vi "Get DAQ Time Array from Waveform.vi"(8 "error in (no error)":errorcluster, 9 "DAQ dt":dbl format="%#_13g", 10 "DAQ Average Number of Points":dbl format="%#_13g", 11 "DAQ Number of Samples":dbl) -> (0 "error out":errorcluster, 3 "Time Axis":dbl[](array[numeric]))   [LabVIEW 2017, in "File IO.lvlib"]
uses:
  File IO.lvlib
  <vilib>/Analysis/2dsp.llb/Decimate (single shot, DBL).vi
  <vilib>/Analysis/NI_AALPro.lvlib
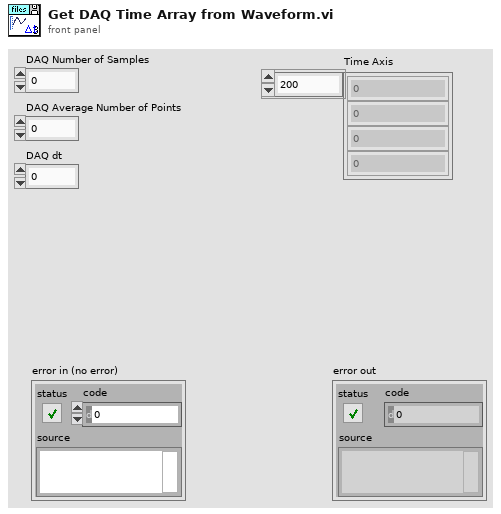
[diagram p1: front panel]
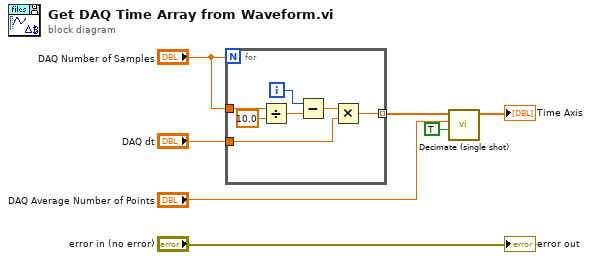
[diagram p0: block diagram]
diagram:
  n1 = for {
    N: "DAQ Number of Samples" -> [_]
    tunnel: "DAQ Number of Samples" -> [w14]
    tunnel: [w9] -> w7 mode=indexing
    tunnel: "DAQ dt" -> [w8]
    i -> [w11]
    n2 = Divide(x=w14, y=10.0) -> (x/y=w12:dbl)
    n3 = Subtract(x=w11, y=w12) -> (x-y=w10:dbl)
    n4 = Multiply(x=w10, y=w8) -> (x*y=w9:dbl)
  }
  n5 = call-poly <vilib>:"Decimate (single shot).vi"("averaging"=TRUE, "decimating factor"="DAQ Average Number of Points", "X"=w7) -> ("Decimated Array"=→"Time Axis":dbl[])  [unwired: 7 in, 1 out]
  "error out" <- "error in (no error)"
